vi "OpenPanel.vi"(3 "CtlRef":refnum<vi>) -> (0 "vi reference":refnum<vi>)   [LabVIEW 2014, in "Panels.lvlib"]
uses:
  Panels.lvlib
panel:
  out "error out":errorcluster
  out "output cluster":cluster{"Top":i16, "Left":i16}
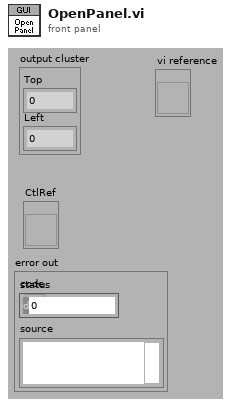
[diagram p1: front panel]
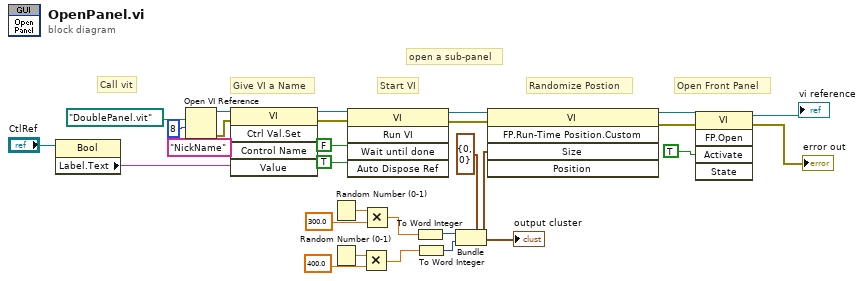
[diagram p0: block diagram]
diagram:
  # "Give VI a Name"
  # "Start VI"
  # "Open Front Panel"
  # "Randomize Postion"
  # "Call vit"
  # "open a sub-panel"
  n1 = property class="Bool"(reference="CtlRef") -> ("Label.Text"=w2:string)  [unwired: 1 in, 2 out]
  n2 = Open VI Reference(vi path=path "DoublePanel.vit", options=8) -> (vi reference=w27:refnum<vi>, error out=w13:errorcluster)  [unwired: 4 in]
  n3 = invoke class="VI" method="Ctrl Val.Set"(reference=w27, error in=w13, "Control Name"="NickName", "Value"=w2) -> (reference out=w10:refnum<vi>, error out=w9:errorcluster)  [unwired: 1 in, 3 out]
  n4 = Random Number (0-1)() -> (number: 0 to 1=w19:dbl)
  n5 = Random Number (0-1)() -> (number: 0 to 1=w21:dbl)
  n6 = invoke class="VI" method="Run VI"(reference=w10, error in=w9, "Wait until done"=FALSE ("Wait Until Done"), "Auto Dispose Ref"=TRUE ("Auto Dispose Reference")) -> (reference out=w8:refnum<vi>, error out=w7:errorcluster)  [unwired: 1 in, 3 out]
  n7 = Multiply(x=w21, y=400.0) -> (x*y=w14:dbl)
  n8 = Multiply(x=w19, y=300.0) -> (x*y=w15:dbl)
  n9 = To Word Integer(number=w15) -> (16bit integer=w17:i16)
  n10 = To Word Integer(number=w14) -> (16bit integer=w16:i16)
  n11 = Bundle(cluster=cluster{"Top":i16, "Left":i16} {"Top"=0, "Left"=0} ("Position"), "Top"=w17, "Left"=w16) -> (w23:cluster{"Top":i16, "Left":i16})
  "output cluster" <- w23
  n12 = invoke class="VI" method="FP.Run-Time Position.Custom"(reference=w8, error in=w7, "Size"=w23) -> (reference out=w6:refnum<vi>, error out=w5:errorcluster)  [unwired: 2 in, 3 out]
  n13 = invoke class="VI" method="FP.Open"(reference=w6, error in=w5, "Activate"=TRUE ("Activate?")) -> (reference out=→"vi reference":refnum<vi>, error out=→"error out":errorcluster)  [unwired: 2 in, 3 out]
